vi "ReCalc_V0.13.vi"() -> ()   [LabVIEW 2014]
uses:
  <vilib>/Utility/miscctls.llb/LVPointTypeDef.ctl
  <vilib>/Utility/NIReport.llb/NI_report.lvclass
  <vilib>/Utility/NIReport.llb/Append Report Text (str wrap).vi
  <vilib>/Utility/xml.llb/Write to XML File(string).vi
  <vilib>/Utility/xml.llb/Read From XML File(string).vi
  <vilib>/Analysis/NI_AALBase.lvlib
  <vilib>/Analysis/NI_AALPro.lvlib
  <vilib>/Analysis/3filter.llb/IIR Filter (DBL).vi
panel:
  out "Überlagerung":bool
  in  "Überlagern":bool
  out "Übersetzung ermitteln aus":T1(ring)
  in  "Datenspeicher":T2
  in  "Speichern":bool
  out "Reifenumfang [m]":dbl=1.222
  out "Getriebe [1:]":dbl=5.343
  out "Zündung [Imp/U]":u8=1
  out "Rolle [Inkr/U]":u16=200
  out "Luftdruck [mbar]":dbl=1013.0
  out "Luftfeuchtigkeit [%]":dbl=50.0
  out "Lufttemperatur [°C]":dbl=20.0
  in  "Berechnen":bool
  in  "Stopp":bool
  in  "Rollenträgheit [kgm²]":dbl=0.402
  in  "Polynom":u8=15
  in  "Gl. Mittelwert":u8=35
  in  "Differenzenquotient":u8=12
  in  "n vom Gas [1/min]":dbl=5000.0
  out "Rollenumfang [m]":dbl=0.613 format="%.3f"
  out "Datum, Zeit":string
  out "Untersetzung aus:":dbl=2.68 format="%.2f"
  in  "Drucken":bool
  out "Pmax":string
  out "Ergebnis":string
  out "Fahrzeugdaten":string
  out "XY-Graph":cluster{dbl[], dbl[]}[](graph)
  in  "Öffnen":bool
  out "korr":dbl
  out "[s]":dbl=5.0
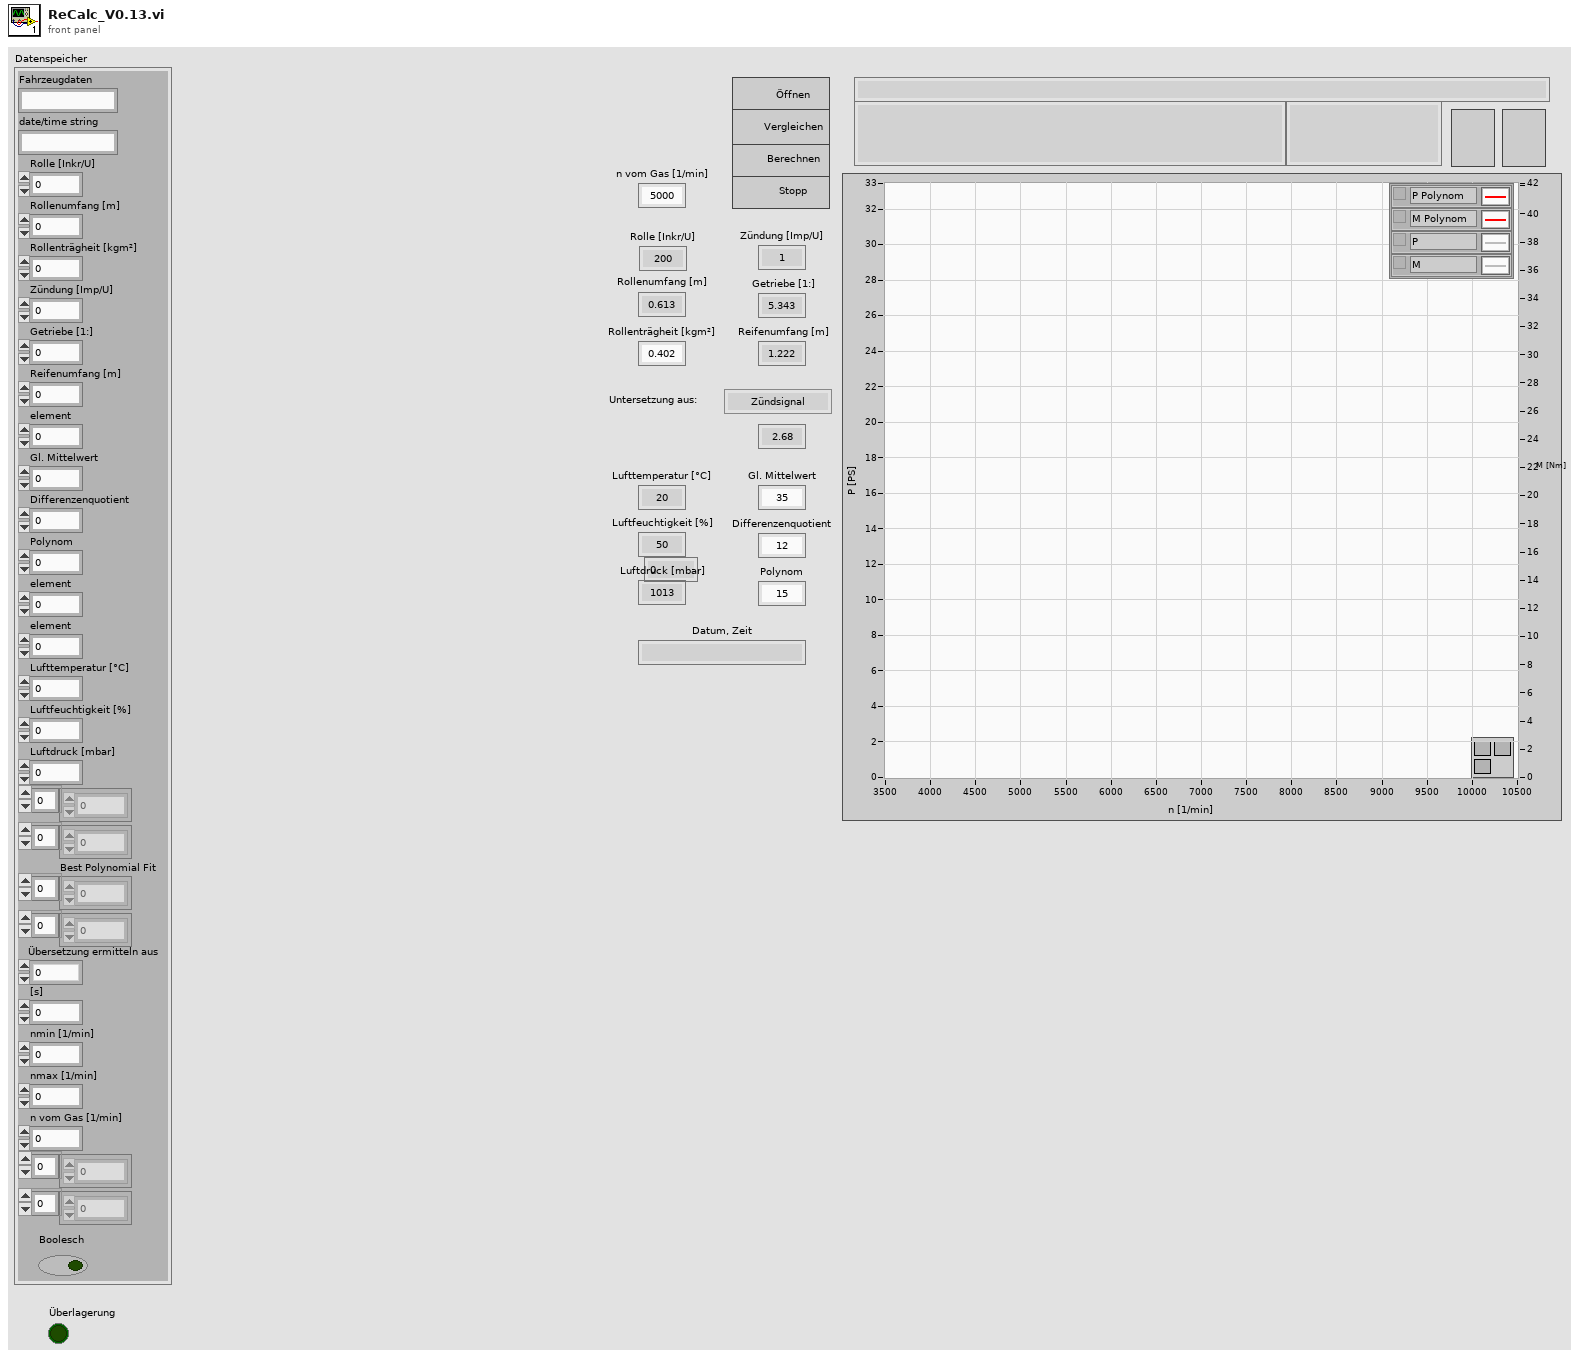
[diagram p1: front panel]
types:
  T1 = enum8{"Zündsignal", "Getriebe & Reifen", "nKuWe / nRolle :"}
  T2 = cluster{"Fahrzeugdaten":string, "date/time string":string, "Rolle [Inkr/U]":u16, "Rollenumfang [m]":dbl, "Rollenträgheit [kgm²]":dbl, "Zündung [Imp/U]":u8, "Getriebe [1:]":dbl, "Reifenumfang [m] ":dbl, "element":dbl, "Gl. Mittelwert":u8, "Differenzenquotient":u8, "Polynom":u8, "element":dbl, "element":dbl, "Lufttemperatur [°C]":dbl, "Luftfeuchtigkeit [%]":dbl, "Luftdruck [mbar]":dbl, dbl[], dbl[], "Best Polynomial Fit":dbl[], dbl[], "Übersetzung ermitteln aus":u8, "[s]":dbl, "nmin [1/min]":dbl, "nmax [1/min]":dbl, "n vom Gas [1/min]":dbl, dbl[], i32[], "Boolesch":bool}
  T3 = typedef "LVPointTypeDef.ctl" = cluster{"Horizontal":i16, "Vertical":i16}
  T4 = enum16{"Kleinste Quadrate", "Kleinestes absolutes Reiduum", "Biquadrat"}
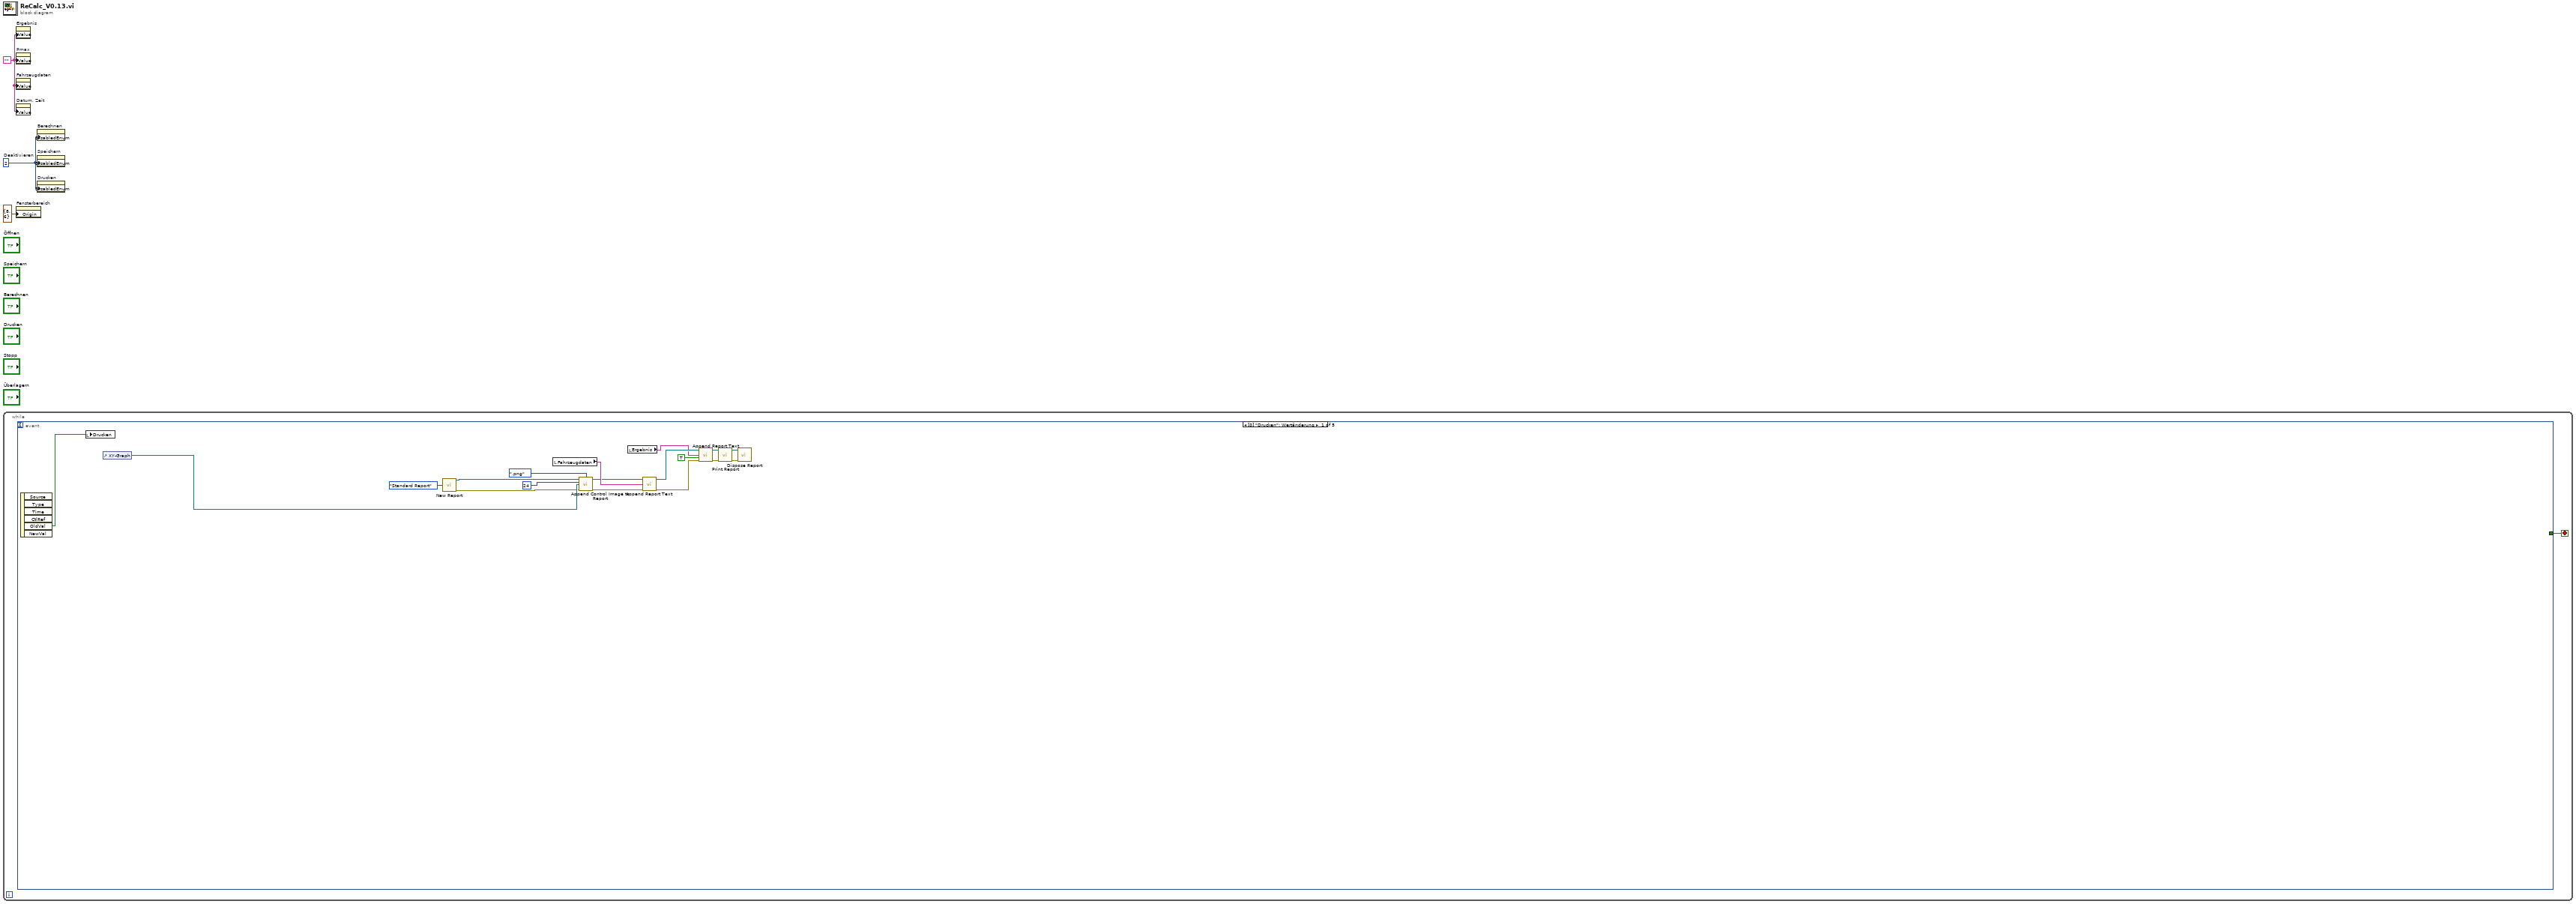
[diagram p0: block diagram]
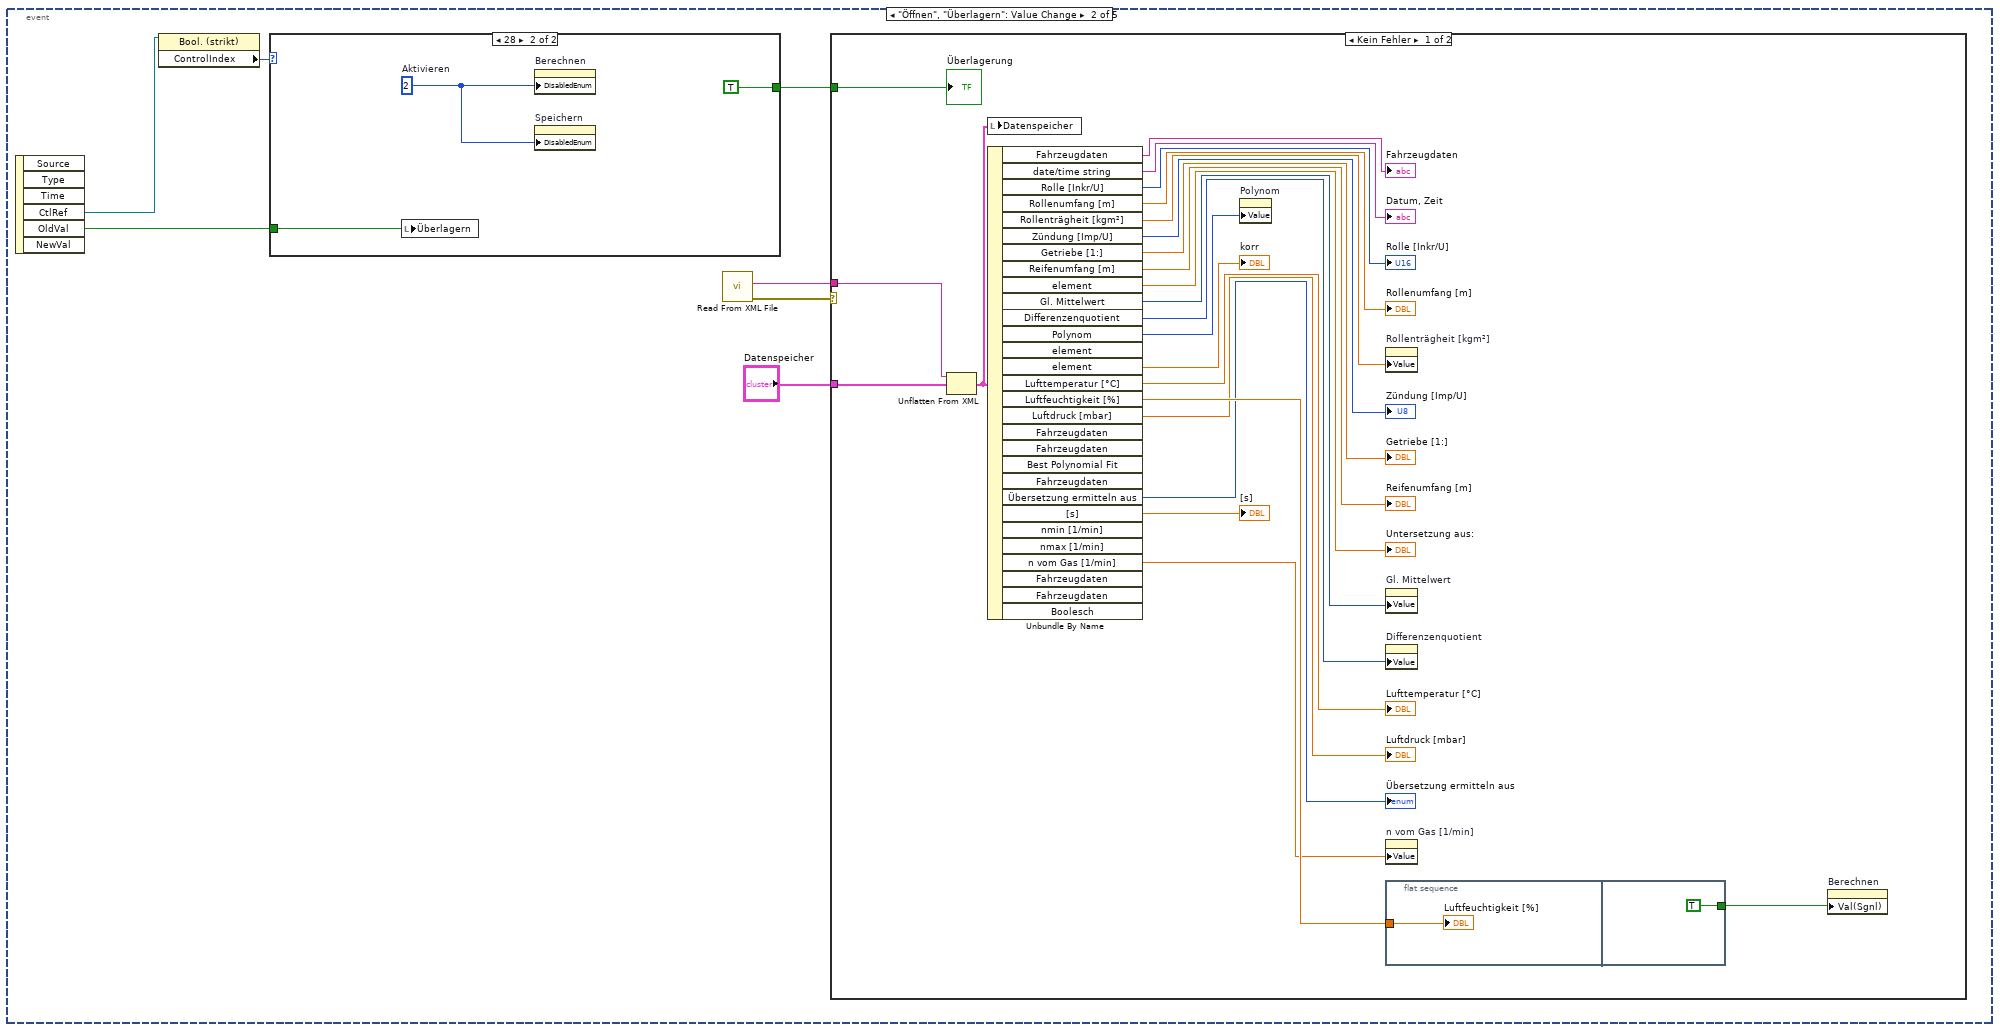
[diagram p2: hidden frame]
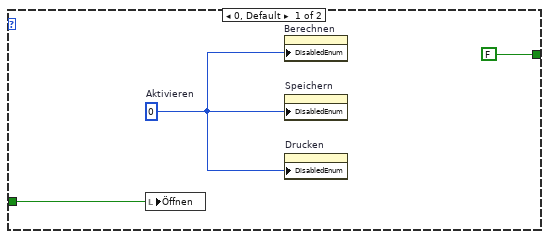
[diagram p3: hidden frame]
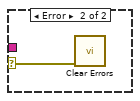
[diagram p4: hidden frame]
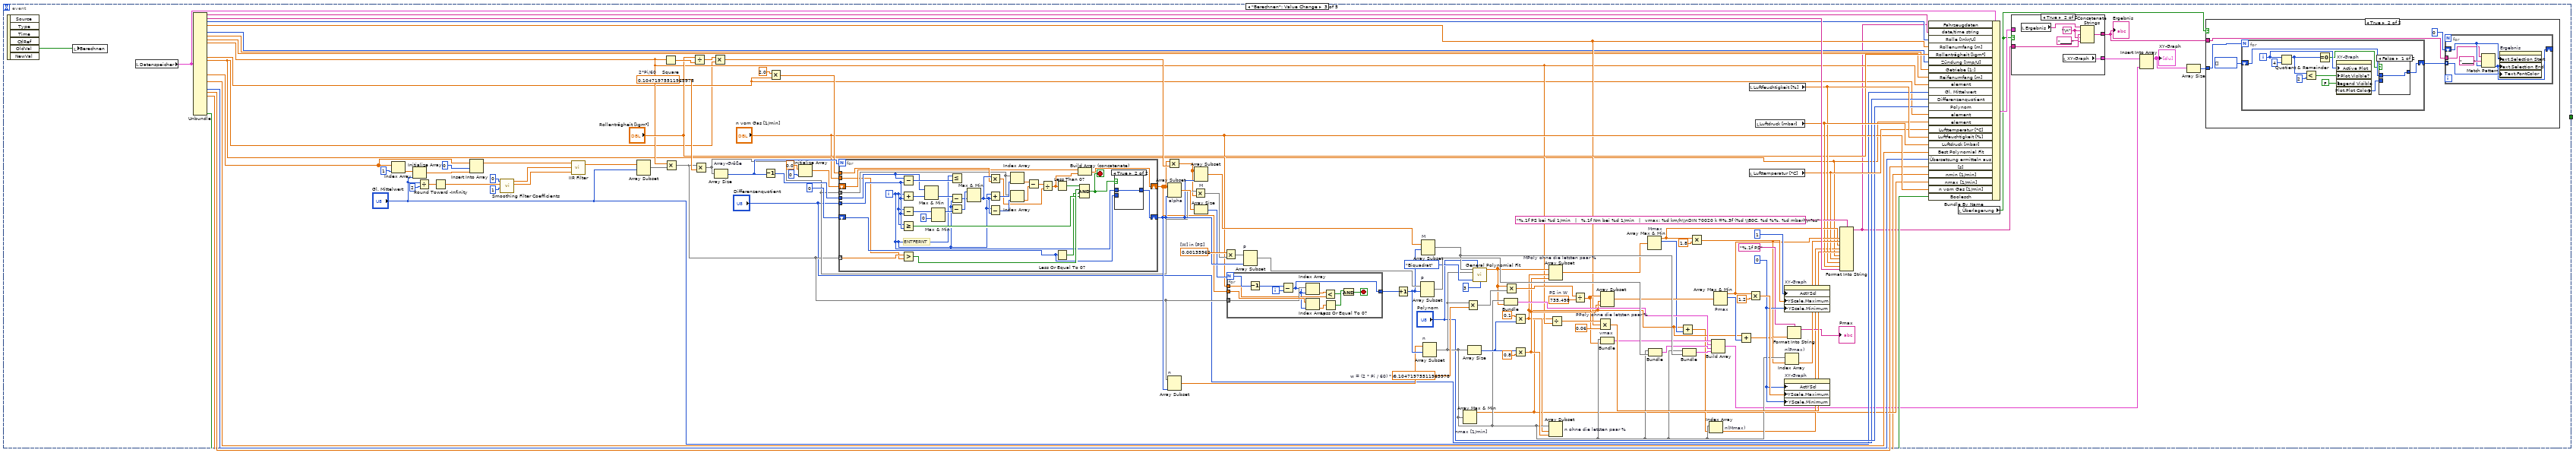
[diagram p5: hidden frame]
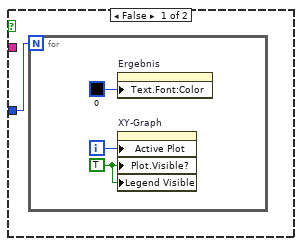
[diagram p6: hidden frame]
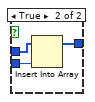
[diagram p7: hidden frame]
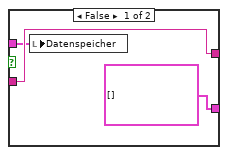
[diagram p8: hidden frame]
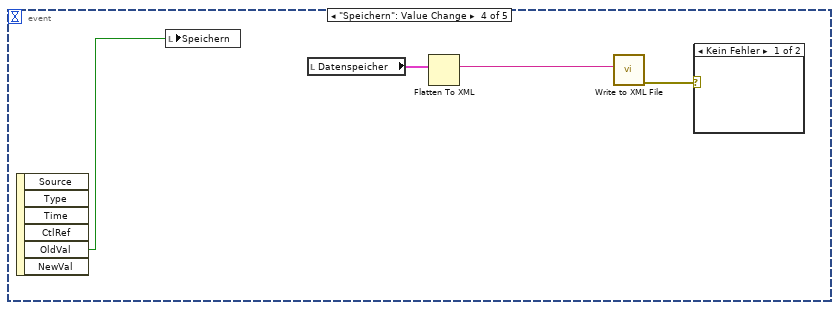
[diagram p10: hidden frame]
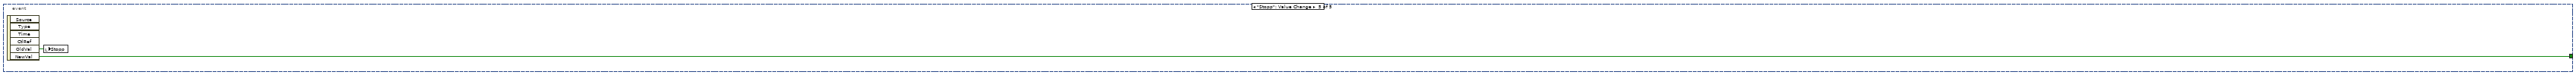
[diagram p12: hidden frame]
diagram:
  w1 = 2  # Deaktivieren
  w3 = ""
  n1 = while {
    stop <- w4 stop-if-true
    n2 = event shown="[0] \"Drucken\": Wertänderung" {
      selector: _ -> [_ _ _ _ _]
      dyn-events: _ -> [_ _ _ _ _]
      timeout: _ -> [_ _ _ _ _]
      tunnel: [_ _ _ _ w269] -> w4
      event "Drucken": Value Change {
        n3 = event-data() -> ("OldVal"=w22:bool)  [unwired: 1 in, 5 out]
        n4 = local write "Drucken"(w22) -> ()
        n5 = control-ref of="XY-Graph"() -> (w21:refnum<vi>)
        n6 = call <vilib>:"New Report.vi"("report type"=enum16{"Standard Report", "HTML"}."Standard Report") -> ("report out"=w19:refnum<class "NI_report.lvclass">, "error out"=w18:errorcluster)  [unwired: 13 in]
        n7 = local read "Fahrzeugdaten"() -> (w20:string)
        n8 = call-dynamic "Append Control Image to Report.vi"("report in"=w19, "image file type (.jpg)"=enum16{".jpg", ".png"}.".png", "image depth"=24, "ctrl reference"=w21, "error in (no error)"=w18) -> ("report out"=w14:refnum<class "NI_report.lvclass">, "error out"=w15:errorcluster)  [unwired: 7 in, 2 out]
        n9 = local read "Ergebnis"() -> (w9:string)
        n10 = call-poly <vilib>:"Append Report Text.vi"("report in"=w14, "text"=w20, "error in (no error)"=w15) -> ("report out"=w13:refnum<class "NI_report.lvclass">, "error out"=w12:errorcluster)  [unwired: 9 in, 2 out]
        n11 = call-poly <vilib>:"Append Report Text.vi"("report in"=w13, "text"=w9, "append on new line? (F)"=TRUE, "error in (no error)"=w12) -> ("report out"=w8:refnum<class "NI_report.lvclass">, "error out"=w7:errorcluster)  [unwired: 8 in, 2 out]
        n12 = call-dynamic "Print Report.vi"("report in"=w8, "error in (no error)"=w7) -> ("report out"=w16:refnum<class "NI_report.lvclass">, "error out"=w17:errorcluster)  [unwired: 12 in]
        n13 = call-dynamic "Dispose Report.vi"("report in"=w16, "error in (no error)"=w17) -> ()  [unwired: 13 in, 1 out]
      }
      event "Öffnen", "Überlagern": Value Change {
        n14 = event-data() -> ("CtlRef"=w26:refnum<vi>, "OldVal"=w24:bool)  [unwired: 1 in, 4 out]
        n15 = property class="Bool. (strikt)"(reference=w26) -> ("ControlIndex"=w25:i32)  [unwired: 1 in, 2 out]
        n16 = case shown="28" w25 {
          tunnel: w24 -> [w32 w35]
          tunnel: [FALSE ("Überlagerung") TRUE ("Überlagerung")] -> w23
          frame 0, Default {
            w30 = 0  # Aktivieren
            n17 = local write "Öffnen"(w32) -> ()
            n18 = property on="Berechnen" class="Bool. (strikt)"("DisabledEnum"=w30) -> ()  [unwired: 2 in, 2 out]
            n19 = property on="Speichern" class="Bool. (strikt)"("DisabledEnum"=w30) -> ()  [unwired: 2 in, 2 out]
            n20 = property on="Drucken" class="Bool. (strikt)"("DisabledEnum"=w30) -> ()  [unwired: 2 in, 2 out]
          }
          frame 28 {
            w33 = 2  # Aktivieren
            n21 = local write "Überlagern"(w35) -> ()
            n22 = property on="Berechnen" class="Bool. (strikt)"("DisabledEnum"=w33) -> ()  [unwired: 2 in, 2 out]
            n23 = property on="Speichern" class="Bool. (strikt)"("DisabledEnum"=w33) -> ()  [unwired: 2 in, 2 out]
          }
        }
        n24 = call-poly <vilib>:"Read From XML File.vi"() -> ("error out"=w27:errorcluster, "XML Elements"=w29:string)  [unwired: 9 in, 1 out]
        n25 = case shown="Kein Fehler" w27 {
          selector: w27 -> [_ w62]
          tunnel: w29 -> [w59 _]
          tunnel: "Datenspeicher" -> [w58 _]
          tunnel: w23 -> [w36 _]
          frame No Error {
            n26 = Unflatten From XML(xml string=w59, type=w58) -> (value=w37:T2)  [unwired: 1 in, 1 out]
            n27 = local write "Datenspeicher"(w37) -> ()
            n28 = Unbundle By Name(w37) -> ("Fahrzeugdaten"=→"Fahrzeugdaten":string, "date/time string"=→"Datum, Zeit":string, "Rolle [Inkr/U]"=→"Rolle [Inkr/U]":u16, "Rollenumfang [m]"=→"Rollenumfang [m]":dbl, "Rollenträgheit [kgm²]"=w53:dbl, "Zündung [Imp/U]"=→"Zündung [Imp/U]":u8, "Getriebe [1:]"=→"Getriebe [1:]":dbl, "Reifenumfang [m]"=→"Reifenumfang [m]":dbl, "element"=→"Untersetzung aus:":dbl, "Gl. Mittelwert"=w50:u8, "Differenzenquotient"=w49:u8, "Polynom"=w48:u8, "element"=→"korr":dbl, "Lufttemperatur [°C]"=→"Lufttemperatur [°C]":dbl, "Luftfeuchtigkeit [%]"=w46:dbl, "Luftdruck [mbar]"=→"Luftdruck [mbar]":dbl, "Übersetzung ermitteln aus"=→"Übersetzung ermitteln aus":u8, "[s]"=→"[s]":dbl, "n vom Gas [1/min]"=w41:dbl)  [unwired: 10 out]
            n29 = property on="Polynom" class="DigWert (strikt)"("Value"=w48) -> ()  [unwired: 2 in, 2 out]
            n30 = property on="Rollenträgheit [kgm²]" class="DigWert (strikt)"("Value"=w53) -> ()  [unwired: 2 in, 2 out]
            n31 = property on="Gl. Mittelwert" class="DigWert (strikt)"("Value"=w50) -> ()  [unwired: 2 in, 2 out]
            n32 = property on="Differenzenquotient" class="DigWert (strikt)"("Value"=w49) -> ()  [unwired: 2 in, 2 out]
            n33 = property on="n vom Gas [1/min]" class="DigWert (strikt)"("Value"=w41) -> ()  [unwired: 2 in, 2 out]
            n34 = flat-sequence {
              tunnel: w46 -> [w60]
              tunnel: [TRUE] -> w38
              frame #0 {
                "Luftfeuchtigkeit [%]" <- w60
              }
              frame #1 {
              }
            }
            n35 = property on="Berechnen" class="Bool. (strikt)"("Val(Sgnl)"=w38) -> ()  [unwired: 2 in, 2 out]
            "Überlagerung" <- w36
          }
          frame Error {
            n36 = call <vilib>:"Clear Errors.vi"("error in (no error)"=w62) -> ()  [unwired: 5 in, 2 out]
          }
        }
      }
      event "Berechnen": Value Change {
        w140 = 0
        w148 = 735.498  # PS in W
        w153 = 0.10471975511965978  # w = (2 * Pi / 60) * n
        w164 = 0.00135962  # [W] in [PS]
        w173 = 0.10471975511965978  # 2*Pi/60
        n37 = event-data() -> ("OldVal"=w69:bool)  [unwired: 1 in, 5 out]
        n38 = local write "Berechnen"(w69) -> ()
        n39 = local read "Datenspeicher"() -> (w96:T2)
        n40 = Unbundle(w96) -> ("Fahrzeugdaten"=w91:string, "date/time string"=w180:string, "Rolle [Inkr/U]"=w92:u16, "Rollenumfang [m]"=w82:dbl, "Zündung [Imp/U]"=w81:u8, "Getriebe [1:]"=w80:dbl, "Reifenumfang [m]"=w79:dbl, "element"=w78:dbl, "element"=w77:dbl, "element"=w76:dbl, w179:dbl[], "Best Polynomial Fit"=w75:dbl[], "Übersetzung ermitteln aus"=w83:u8, "[s]"=w72:dbl, "nmin [1/min]"=w73:dbl, "Boolesch"=w86:bool)  [unwired: 13 out]
        n41 = Index Array(array=w179, index=1) -> (element=w102:dbl)
        n42 = Initialize Array(w102, "Gl. Mittelwert") -> (w103:dbl[])
        n43 = Divide(x="Gl. Mittelwert", y=2) -> (x/y=w176:dbl)
        n44 = Round Toward -Infinity(1:w176) -> (0:w175:dbl)
        n45 = Insert Into Array ("In Array einfügen")(array=w179, index=0, new element=w103) -> (w100:dbl[])
        n46 = call <vilib>:"Smoothing Filter Coefficients.vi"("shape"=1, "half-width"=w175, "type"=0) -> ("forward coefficients"=w104:dbl[], "reverse coefficients"=w105:dbl[])  [unwired: 6 in, 1 out]
        n47 = call-poly <vilib>:"IIR Filter.vi"("Forward Coefficients"=w104, "Reverse Coefficients"=w105, "X"=w100) -> ("Filtered X"=w99:dbl[])  [unwired: 1 in, 1 out]
        n48 = Array Subset(array=w99, index="Gl. Mittelwert") -> (w98:dbl[])  [unwired: 1 in]
        n49 = Square(x=w78) -> (x^2=w165:dbl)
        n50 = Multiply(x=w78, y=w98) -> (x*y=w107:dbl[])
        n51 = Divide(x="Rollenträgheit [kgm²]", y=w165) -> (x/y=w162:dbl)
        n52 = Multiply(x=w107, y=w173) -> (x*y=w130:dbl[])
        n53 = Multiply(x=w162, y=w76) -> (x*y=w161:dbl)
        n54 = Array Size "Array-Größe"(array=w130) -> (size(s)=w171:i32)
        n55 = Decrement(x=w171) -> (x-1=w172:i32)
        n56 = Multiply(x=2.0, y=w77) -> (x*y=w170:dbl)
        n57 = Initialize Array(0.0 ("y"), 0) -> (w166:dbl[])
        n58 = for {
          N: w171 -> [_]
          tunnel: "Differenzenquotient" -> [w240]
          tunnel: w130 -> [w247]
          tunnel: w172 -> [w239]
          tunnel: w170 -> [w248]
          shift-right: [w244] -> w129
          shift-left: w166 -> [w245]
          tunnel: w107 -> [w242] mode=indexing
          tunnel: "n vom Gas [1/min]" -> [w231]
          shift-right: [w230] -> w157
          shift-left: 0 -> [w233]
          i -> [w234]
          stop <- w232 stop-if-true
          # "ENTFERNT"
          n59 = Subtract(x=w239, y=w240) -> (x-y=w241:i32)
          n60 = Add(x=w234, y=w240) -> (x+y=w255:i32)
          n61 = Subtract(x=w234, y=w240) -> (x-y=w261:i32)
          n62 = Greater Or Equal?(x=w234, y=w240) -> (x >= y?=w237:bool)
          n63 = Greater?(x=w242, y=w231) -> (0:w243:bool)
          n64 = Max & Min(x=w239, y=w255) -> (min(x,y)=w256:i32)  [unwired: 1 out]
          n65 = Max & Min(x=w261, y=0) -> (max(x,y)=w259:i32)  [unwired: 1 out]
          n66 = Less Or Equal?(x=w234, y=w241) -> ()  [unwired: 1 out]
          n67 = Subtract(x=w256, y=w234) -> (x-y=w257:i32)
          n68 = Subtract(x=w234, y=w259) -> (x-y=w258:i32)
          n69 = Max & Min(x=w258, y=w257) -> (min(x,y)=w249:i32)  [unwired: 1 out]
          n70 = Multiply(x=w249, y=w248) -> (x*y=w246:dbl)
          n71 = Add(x=w234, y=w249) -> (x+y=w254:i32)
          n72 = Subtract(x=w234, y=w249) -> (x-y=w253:i32)
          n73 = Index Array(array=w247, index=w254) -> (element=w251:dbl)
          n74 = Index Array(array=w247, index=w253) -> (element=w252:dbl)
          n75 = Subtract(x=w251, y=w252) -> (x-y=w250:dbl)
          n76 = Divide(x=w250, y=w246) -> (x/y=w238:dbl)
          n77 = Less Than 0?(x=w238) -> (x < 0?=w236:bool)
          n78 = Less Or Equal To 0?(x=w233) -> (x <= 0?=w235:bool)
          n79 = Build Array (concatenate)(w245, w238) -> (w244:dbl[])
          n80 = Compound Arithmetic op=AND(w236, w243, w235, w237) -> (w232:bool)
          n81 = case shown="True" w232 {
            tunnel: w234 -> [_ w263]
            tunnel: [w262 w263] -> w230
            tunnel: w233 -> [w262 _]
            frame False {
            }
            frame True {
            }
          }
        }
        n82 = Multiply(x=w129, y=w161) -> (x*y=w127:dbl[])
        n83 = Array Subset "alpha"(array=w129, length=w157) -> (w159:dbl[])  [unwired: 1 in]
        n84 = Array Subset "n"(array=w107, length=w157) -> (w106:dbl[])  [unwired: 1 in]
        n85 = Multiply(x=w130, y=w127) -> (x*y=w163:dbl[])
        n86 = Array Subset "M"(array=w127, length=w157) -> (w128:dbl[])  [unwired: 1 in]
        n87 = Array Size(array=w159) -> (size(s)=w156:i32)
        n88 = Multiply(x=w164, y=w163) -> (x*y=w158:dbl[])
        n89 = for {
          N: w156 -> [w229]
          tunnel: w129 -> [w226]
          tunnel: w107 -> [w223]
          tunnel: "n vom Gas [1/min]" -> [w220]
          tunnel: [w218] -> w155
          i -> [w224]
          stop <- w219 stop-if-true
          n90 = Decrement(x=w229) -> (x-1=w228:i32)
          n91 = Subtract(x=w228, y=w224) -> (x-y=w218:i32)
          n92 = Index Array(array=w223, index=w218) -> (element=w222:dbl)
          n93 = Index Array(array=w226, index=w218) -> (element=w227:dbl)
          n94 = Less?(x=w222, y=w220) -> (x < y?=w221:bool)
          n95 = Less Or Equal To 0?(x=w227) -> (x <= 0?=w225:bool)
          n96 = And(x=w225, y=w221) -> (x .and. y?=w219:bool)
        }
        n97 = Array Subset "P"(array=w158, length=w157) -> (w147:dbl[])  [unwired: 1 in]
        n98 = Increment(x=w155) -> (x+1=w146:i32)
        n99 = Array Subset "P"(array=w147, index=w146) -> (w154:dbl[])  [unwired: 1 in]
        n100 = Array Subset "M"(array=w128, index=w146) -> (w152:dbl[])  [unwired: 1 in]
        n101 = Array Subset "n"(array=w106, index=w146) -> (w115:dbl[])  [unwired: 1 in]
        n102 = Array Max & Min "nmax [1/min]"(array=w115) -> (max value=w74:dbl)  [unwired: 3 out]
        n103 = Multiply(x=w115, y=w153) -> (x*y=w139:dbl[])
        n104 = Array Size(array=w115) -> (size(s)=w117:i32)
        n105 = call <vilib>:"General Polynomial Fit.vi"("Y"=w152, "polynomial order"="Polynom", "X"=w115, "method"=T4."Biquadrat" ("Methode"), "algorithm"=3) -> ("Best Polynomial Fit"=w114:dbl[])  [unwired: 7 in, 3 out]
        n106 = Bundle(w115, "Best Polynomial Fit"=w114) -> (w125:cluster{dbl[], "Best Polynomial Fit":dbl[]})  [unwired: 1 in]
        n107 = Multiply(x=w114, y=w139) -> (x*y=w149:dbl[])
        n108 = Multiply(x=0.1, y=w117) -> (x*y=w110:dbl)
        n109 = Multiply(x=w117, y=0.8) -> (x*y=w118:dbl)
        n110 = Array Subset "MPoly ohne die letzten paar %"(array=w114, index=w110, length=w118) -> (w119:dbl[])
        n111 = Array Subset "n ohne die letzten paar %"(array=w115, index=w110, length=w118) -> ()  [unwired: 1 out]
        n112 = Divide(x=w74, y=w78) -> (x/y=w138:dbl)
        n113 = Divide(x=w149, y=w148) -> (x/y=w113:dbl[])
        n114 = Array Subset "PPoly ohne die letzten paar %"(array=w113, index=w110, length=w118) -> (w120:dbl[])
        n115 = Compound Arithmetic op=MULTIPLY "vmax"(w138, w82, 0.06) -> (w135:dbl)
        n116 = Bundle(w115, w113) -> (w126:cluster{dbl[], dbl[]})  [unwired: 1 in]
        n117 = Array Max & Min "Mmax"(array=w119) -> (max value=w132:dbl, max index (indices)=w111:i32)  [unwired: 2 out]
        n118 = Bundle(w115, w154) -> (w124:cluster{dbl[], dbl[]})  [unwired: 1 in]
        n119 = Add(x=w110, y=w111) -> (x+y=w109:dbl)
        n120 = Bundle(w115, w152) -> (w123:cluster{dbl[], dbl[]})  [unwired: 1 in]
        n121 = Multiply(x=w132, y=1.8) -> (x*y=w141:dbl)
        n122 = Index Array "n(Mmax)"(array=w115, index=w109) -> (element=w84:dbl)
        n123 = Build Array(w126, w125, w124, w123) -> (w65:cluster{dbl[], "Best Polynomial Fit":dbl[]}[])
        n124 = Array Max & Min "Pmax"(array=w120) -> (max value=w133:dbl, max index (indices)=w112:i32)  [unwired: 2 out]
        n125 = Add(x=w110, y=w112) -> (x+y=w108:dbl)
        n126 = Multiply(x=w133, y=1.2) -> (x*y=w142:dbl)
        n127 = local read "Luftfeuchtigkeit [%]"() -> (w94:dbl)
        n128 = local read "Lufttemperatur [°C]"() -> (w93:dbl)
        n129 = local read "Luftdruck [mbar]"() -> (w95:dbl)
        n130 = property on="XY-Graph" class="XYGraph (strikt)"("ActYScl"=1, "YScale.Maximum"=w141, "YScale.Minimum"=w140) -> ()  [unwired: 2 in, 2 out]
        n131 = property on="XY-Graph" class="XYGraph (strikt)"("ActYScl"=w140, "YScale.Maximum"=w142, "YScale.Minimum"=w140) -> ()  [unwired: 2 in, 2 out]
        n132 = Index Array "n(Pmax)"(array=w115, index=w108) -> (element=w136:dbl)
        n133 = Format Into String(format string="%.1f PS" ("Format-String"), w133) -> (resulting string=→"Pmax":string)  [unwired: 2 in, 1 out]
        n134 = Format Into String(format string="%.1f PS bei %d 1/min   |   %.1f Nm bei %d 1/min   |   vmax: %d km/h\\nDIN 70020 k =%.3f (%d \\B0C, %d %%, %d mbar)\\n%s" ("Format-String"), w133, w136, w132, w84, w135, w76, w93, w94, w95, w180) -> (resulting string=w71:string)  [unwired: 2 in, 1 out]
        n135 = Bundle By Name(cluster=w96, "Fahrzeugdaten"=w71, "date/time string"=w91, "Rolle [Inkr/U]"=w92, "Rollenumfang [m]"=w82, "Rollenträgheit [kgm²]"="Rollenträgheit [kgm²]", "Zündung [Imp/U]"=w81, "Getriebe [1:]"=w80, "Reifenumfang [m]"=w79, "element"=w78, "Gl. Mittelwert"="Gl. Mittelwert", "Differenzenquotient"="Differenzenquotient", "Polynom"="Polynom", "element"=w77, "element"=w76, "Lufttemperatur [°C]"=w93, "Luftfeuchtigkeit [%]"=w94, "Luftdruck [mbar]"=w95, "Best Polynomial Fit"=w75, "Übersetzung ermitteln aus"=w83, "[s]"=w72, "nmin [1/min]"=w73, "nmax [1/min]"=w74, "n vom Gas [1/min]"="n vom Gas [1/min]", "Boolesch"=w86) -> (w67:T2)
        n136 = local read "Überlagerung"() -> (w66:bool)
        n137 = case shown="True" w66 {
          tunnel: [cluster{dbl[], dbl[]}[] [] ("XY-Graph") w217] -> w64
          tunnel: w71 -> [w210 w214]
          tunnel: [w210 w215] -> w63
          tunnel: w67 -> [w209 _]
          frame False {
            n138 = local write "Datenspeicher"(w209) -> ()
          }
          frame True {
            w212 = "\n"
            n139 = local read "Ergebnis"() -> (w216:string)
            n140 = local read "XY-Graph"() -> (w217:cluster{dbl[], dbl[]}[])
            n141 = Concatenate Strings(w216, w212, "_____" ("String"), w212, w214) -> (w215:string)
          }
        }
        "Ergebnis" <- w63
        n142 = Insert Into Array(array=w64, new element=w65) -> (w68:cluster{dbl[], dbl[]}[])  [unwired: 1 in]
        "XY-Graph" <- w68
        n143 = Array Size(array=w68) -> (size(s)=w70:i32)
        n144 = case shown="True" w66 {
          tunnel: w70 -> [w181 w189]
          tunnel: w63 -> [_ w185]
          frame False {
            n145 = for {
              N: w181 -> [_]
              i -> [w184]
              w183 = TRUE ("Plot.Sichtbar")
              n146 = property on="Ergebnis" class="Str"("Text.Font:Color"=u32 0) -> ()  [unwired: 2 in, 2 out]
              n147 = property on="XY-Graph" class="XYGraph (strikt)"("Active Plot"=w184, "Plot.Visible?"=w183, "Legend Visible"=w183) -> ()  [unwired: 2 in, 2 out]
            }
          }
          frame True {
            n148 = for {
              N: w189 -> [_]
              shift-right: [w197] -> w186
              shift-left: u32[] [] -> [w196]
              i -> [w203]
              n149 = Quotient & Remainder(x=w203, y=4) -> (x-y*floor(x/y)=w199:i32)  [unwired: 1 out]
              n150 = Less?(x=w199, y=2) -> (x < y?=w202:bool)
              n151 = Equal To 0?(x=w199) -> (x = 0?=w195:bool)
              n152 = property on="XY-Graph" class="XYGraph (strikt)"("Active Plot"=w203, "Plot.Visible?"=w202, "Legend Visible"=FALSE ("Legende:Sichtbar")) -> ("Plot.Plot Color"=w198:u32)  [unwired: 2 in, 2 out]
              n153 = case shown="False" w195 {
                tunnel: w198 -> [_ w208]
                tunnel: [w205 w207] -> w197
                tunnel: w196 -> [w205 w206]
                frame False {
                }
                frame True {
                  n154 = Insert Into Array(array=w206, new element=w208) -> (w207:u32[])  [unwired: 1 in]
                }
              }
            }
            n155 = for {
              shift-right: [w192] -> _
              shift-left: 0 -> [w191]
              tunnel: w186 -> [w193] mode=indexing
              tunnel: w185 -> [w190]
              n156 = Match Pattern(string=w190, regular expression="_____" ("String"), offset (0)=w191) -> (offset past match=w192:i32)  [unwired: 3 out]
              n157 = property on="Ergebnis" class="Str"("Text.Selection Start"=w191, "Text.Selection End"=w192, "Text.FontColor"=w193) -> ()  [unwired: 2 in, 2 out]
            }
          }
        }
      }
      event "Speichern": Value Change {
        n158 = event-data() -> ("OldVal"=w264:bool)  [unwired: 1 in, 5 out]
        n159 = local write "Speichern"(w264) -> ()
        n160 = local read "Datenspeicher"() -> (w265:T2)
        n161 = Flatten To XML(anything=w265) -> (xml string=w267:string)
        n162 = call-poly <vilib>:"Write to XML File.vi"("XML Input"=w267) -> ("error out"=w266:errorcluster)  [unwired: 8 in, 2 out]
        n163 = case shown="Kein Fehler" w266 {
          frame No Error {
          }
          frame Error {
          }
        }
      }
      event "Stopp": Value Change {
        n164 = event-data() -> ("OldVal"=w268:bool, "NewVal"=w269:bool)  [unwired: 1 in, 4 out]
        n165 = local write "Stopp"(w268) -> ()
      }
    }
  }
  n166 = property on="Ergebnis" class="Str"("Value"=w3) -> ()  [unwired: 2 in, 2 out]
  n167 = property on="Pmax" class="Str"("Value"=w3) -> ()  [unwired: 2 in, 2 out]
  n168 = property on="Fahrzeugdaten" class="Str"("Value"=w3) -> ()  [unwired: 2 in, 2 out]
  n169 = property on="Datum, Zeit" class="Str"("Value"=w3) -> ()  [unwired: 2 in, 2 out]
  n170 = property on="Fensterbereich" class="Bereich"("Origin"=T3 {"Horizontal"=8, "Vertical"=6}) -> ()  [unwired: 2 in, 2 out]
  n171 = property on="Berechnen" class="Bool. (strikt)"("DisabledEnum"=w1) -> ()  [unwired: 2 in, 2 out]
  n172 = property on="Speichern" class="Bool. (strikt)"("DisabledEnum"=w1) -> ()  [unwired: 2 in, 2 out]
  n173 = property on="Drucken" class="Bool. (strikt)"("DisabledEnum"=w1) -> ()  [unwired: 2 in, 2 out]
